vi "JL_Obtain Time Option From Time in Sec.vi"(0 "Time In Seconds":i16) -> (4 "Fail":bool, 6 "Pass":bool, 8 "Time Option":u8 format="%x")   [LabVIEW 2016]
panel:
  # "All integers are hex"
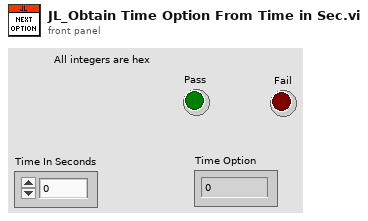
[diagram p1: front panel]
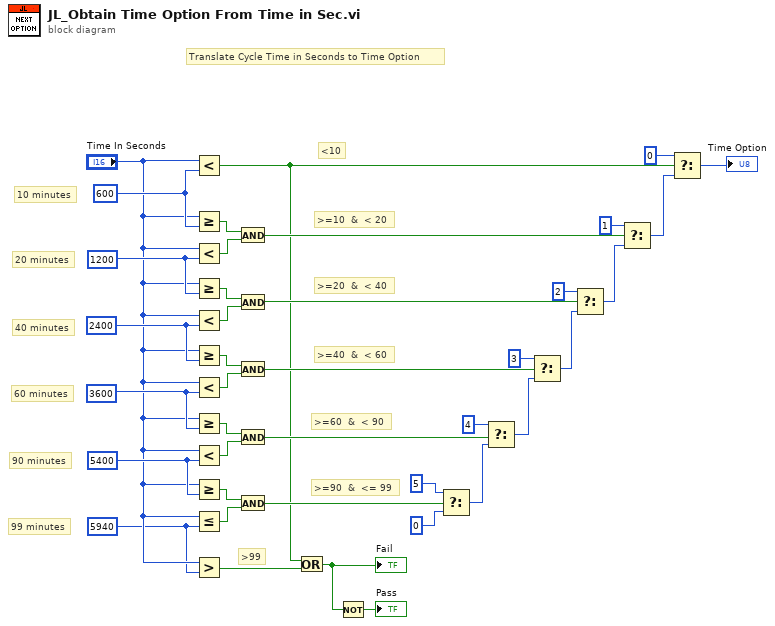
[diagram p0: block diagram]
diagram:
  w6 = i16 5940 ("y")
  w24 = i16 5400 ("y")
  w25 = i16 3600 ("x")
  w28 = i16 2400 ("y")
  w31 = i16 1200 ("y")
  w36 = i16 600 ("y")
  # ">99"
  # ">=90  &  <= 99"
  # ">=60  &  < 90"
  # ">=40  &  < 60"
  # ">=20  &  < 40"
  # ">=10  &  < 20"
  # "<10"
  # "90 minutes"
  # "99 minutes"
  # "60 minutes"
  # "40 minutes"
  # "20 minutes"
  # "10 minutes"
  # "Translate Cycle Time in Seconds to Time Option"
  n1 = Less?(x="Time In Seconds", y=w36) -> (x < y?=w4:bool)
  n2 = Greater Or Equal?(x="Time In Seconds", y=w36) -> (x >= y?=w38:bool)
  n3 = Less?(x="Time In Seconds", y=w31) -> (x < y?=w37:bool)
  n4 = Greater Or Equal?(x="Time In Seconds", y=w31) -> (x >= y?=w35:bool)
  n5 = Less?(x="Time In Seconds", y=w28) -> (x < y?=w34:bool)
  n6 = Greater Or Equal?(x="Time In Seconds", y=w28) -> (x >= y?=w33:bool)
  n7 = Less?(x="Time In Seconds", y=w25) -> (x < y?=w32:bool)
  n8 = Greater Or Equal?(x="Time In Seconds", y=w25) -> (x >= y?=w30:bool)
  n9 = Less?(x="Time In Seconds", y=w24) -> (x < y?=w29:bool)
  n10 = Greater Or Equal?(x="Time In Seconds", y=w24) -> (x >= y?=w27:bool)
  n11 = Less Or Equal?(x="Time In Seconds", y=w6) -> (x <= y?=w26:bool)
  n12 = Greater?(x="Time In Seconds", y=w6) -> (0:w5:bool)
  n13 = And(x=w38, y=w37) -> (x .and. y?=w22:bool)
  n14 = And(x=w35, y=w34) -> (x .and. y?=w19:bool)
  n15 = And(x=w33, y=w32) -> (x .and. y?=w10:bool)
  n16 = And(x=w30, y=w29) -> (x .and. y?=w9:bool)
  n17 = And(x=w27, y=w26) -> (x .and. y?=w8:bool)
  n18 = Or(x=w4, y=w5) -> (x .or. y?=w2:bool)
  "Fail" <- w2
  n19 = Not(x=w2) -> (.not. x?=→"Pass":bool)
  n20 = Select(t=u8 5, s=w8, f=u8 0) -> (s? t:f=w11:u8)
  n21 = Select(t=u8 4, s=w9, f=w11) -> (s? t:f=w12:u8)
  n22 = Select(t=u8 3, s=w10, f=w12) -> (s? t:f=w13:u8)
  n23 = Select(t=u8 2, s=w19, f=w13) -> (s? t:f=w20:u8)
  n24 = Select(t=u8 1, s=w22, f=w20) -> (s? t:f=w23:u8)
  n25 = Select(t=u8 0, s=w4, f=w23) -> (s? t:f=→"Time Option":u8)
